vi "niUSRP Rx Continuous Lab.vi"() -> ()   [LabVIEW 2014]
uses:
  <instrlib>/niUSRP/niUSRP Fetch Rx Data (CDB WDT).vi
  <vilib>/measure/maspectr.llb/FFT Power Spectrum and PSD for 1 Chan (CDB).vi
  <vilib>/measure/NI_MAPro.lvlib
panel:
  out "Waveform Graph":dbl[](graph)
  in  "Stop Button":bool
  out "Frequency Plot":cluster{"f0":dbl, "df":dbl, "magnitude":dbl[]}(graph)
  out "IQ Plot":waveform(dbl)[](graph)
  in  "device name":refnum<k15>="192.168.10.2"
  in  "Active Antenna":string(combo)="RX1"
  in  "samples / frame":i64=1000
  out "Error Out":errorcluster
  out "Gain [dB] (actual)":dbl format="%#.6p"
  out "Carrier Frequency \n[Hz] (actual)":dbl=2450000000.0 format="%#.6p"
  out "IQ Sampling\nRate [s/sec] (actual)":dbl=10000000.0 format="%#.6p"
  in  "Gain [dB]":dbl format="%#.6p"
  in  "Carrier\nFrequency [Hz]":dbl=915000000.0 format="%#.6p"
  in  "IQ Sampling\nRate [s/sec]":dbl=10000000.0 format="%#.6p"
  # "IQ Receiver"
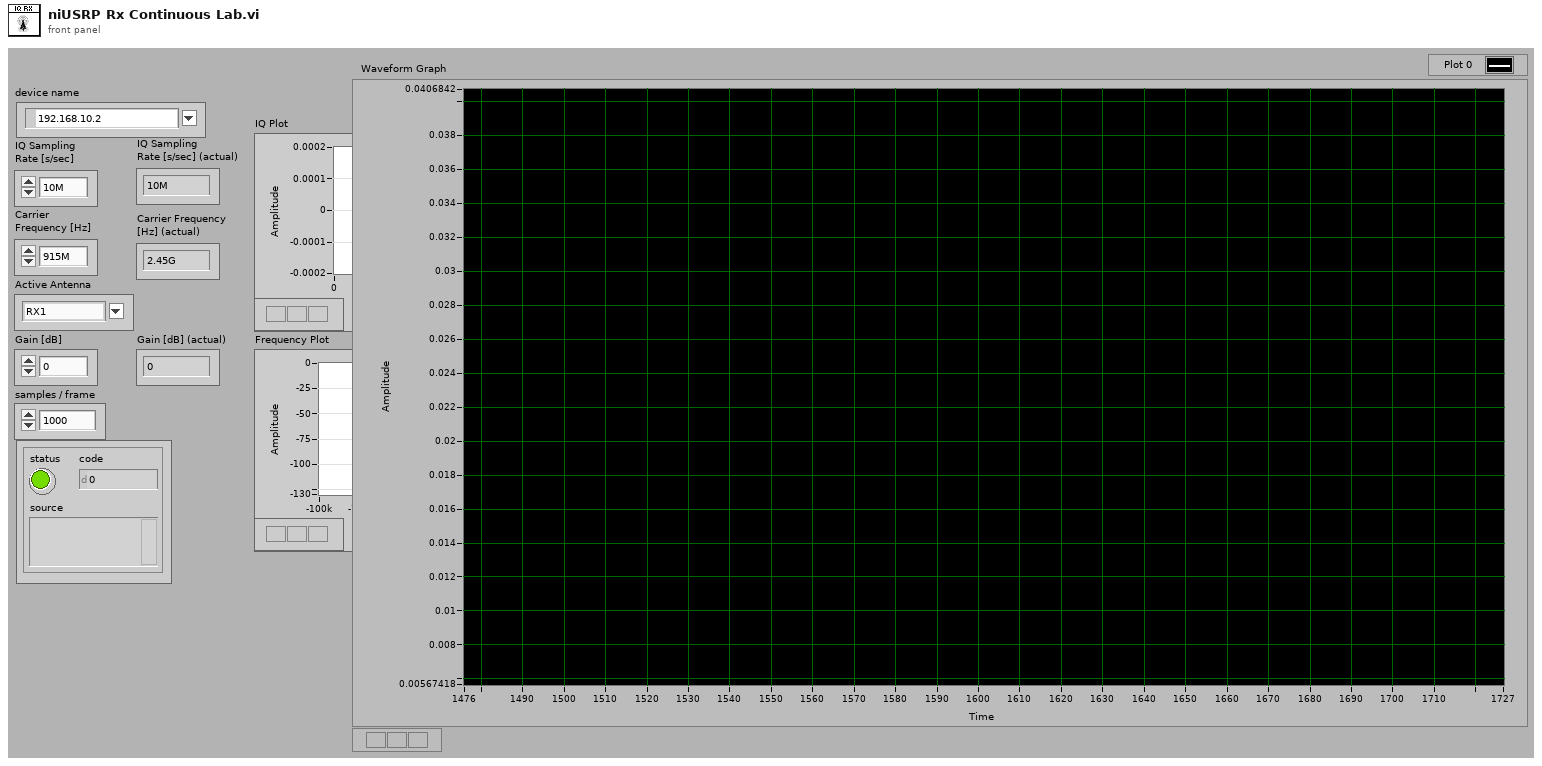
[diagram p1: front panel]
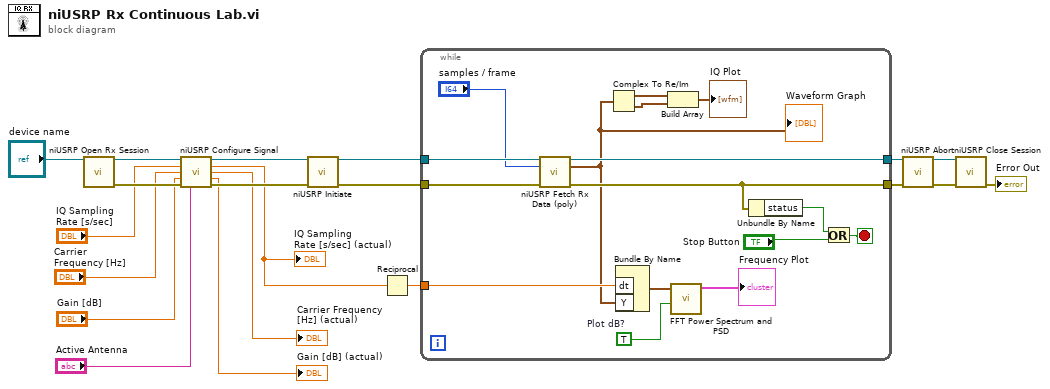
[diagram p0: block diagram]
diagram:
  n1 = call <instrlib>:"niUSRP Open Rx Session.vi"("device names"="device name") -> ("session handle out"=w19:refnum<k15>, "error out"=w18:errorcluster)  [unwired: 13 in]
  n2 = call <instrlib>:"niUSRP Configure Signal.vi"("session handle"=w19, "IQ rate"="IQ Sampling\nRate [s/sec]", "carrier frequency"="Carrier\nFrequency [Hz]", "gain"="Gain [dB]", "error in (no error)"=w18, "active antenna"="Active Antenna") -> ("session handle out"=w8:refnum<k15>, "coerced IQ rate"=w3:dbl, "coerced carrier frequency"=→"Carrier Frequency \n[Hz] (actual)":dbl, "coerced gain"=→"Gain [dB] (actual)":dbl, "error out"=w10:errorcluster)  [unwired: 5 in]
  "IQ Sampling\nRate [s/sec] (actual)" <- w3
  n3 = call <instrlib>:"niUSRP Initiate.vi"("session handle"=w8, "error in (no error)"=w10) -> ("session handle out"=w14:refnum<k15>, "error out"=w13:errorcluster)  [unwired: 12 in]
  n4 = Reciprocal(x=w3) -> (1/x=w4:dbl)
  n5 = while {
    tunnel: w14 -> [w36]
    tunnel: w13 -> [w35]
    tunnel: w4 -> [w34]
    tunnel: [w29] -> w2
    tunnel: [w28] -> w1
    stop <- w27 stop-if-true
    w30 = TRUE  # Plot dB?
    n6 = call-poly <instrlib>:"niUSRP Fetch Rx Data (poly).vi"("session handle"=w36, "number of samples"="samples / frame", "error in (no error)"=w35) -> ("session handle out"=w29:refnum<k15>, "data"=w21:waveform(cdb), "error out"=w28:errorcluster)  [unwired: 9 in, 1 out]
    "Waveform Graph" <- w21
    n7 = Complex To Re/Im(x + iy=w21) -> (x=w26:waveform(dbl), y=w25:waveform(dbl))
    n8 = Bundle By Name("dt"=w34, "Y"=w21) -> (w31:waveform(cdb))  [unwired: 1 in]
    n9 = Build Array(w26, w25) -> (→"IQ Plot":waveform(dbl)[])
    n10 = call-poly <vilib>:"FFT Power Spectrum and PSD.vi"("dB On (F)"=w30, "time signal"=w31) -> ("Power Spectrum / PSD"=→"Frequency Plot":cluster{"f0":dbl, "df":dbl, "magnitude":dbl[]})  [unwired: 6 in, 3 out]
    n11 = Unbundle By Name(w28) -> ("status"=w33:bool)
    n12 = Or(x=w33, y="Stop Button") -> (x .or. y?=w27:bool)
  }
  n13 = call <instrlib>:"niUSRP Abort.vi"("session handle"=w2, "error in (no error)"=w1) -> ("session handle out"=w16:refnum<k15>, "error out"=w15:errorcluster)  [unwired: 12 in]
  n14 = call <instrlib>:"niUSRP Close Session.vi"("session handle"=w16, "error in (no error)"=w15) -> ("error out"=→"Error Out":errorcluster)  [unwired: 13 in]
